vi "Port D_A Output Level.vi"(7 "Read Value? (F)":bool, 8 "error in (no error)":errorcluster, 9 "Port Output Level (0.000 V)":dbl format="%.3g", 10 "Port (1)":T1=enum."1", 11 "VISA resource name":refnum<visa-resource-name>) -> (0 "error out":errorcluster, 1 "Port Output Level":dbl format="%.3g", 3 "VISA resource name out":refnum<visa-resource-name>)   [LabVIEW 2013, in "SRS SR400.lvlib"]
doc: "<B>PL i { ,v }</B>\n\nThe PL command sets and reads thePORT1 and PORT2 output levels. i=1 or 2 to select PORT1 or PORT 2 and is required. If v is included, the output level is set to v Volts where -10.000 <= v <= 10.000. The resolution is 0.005 V (5 mV). If v is absent, the output level is returned. If the Port output mode is SCAN, the PL command sets and reads the starting value of the level. Changing the level during a scan will cause the level to be set to the new value on the next count period. Note that the scan is not reset. Reading the level during a scan always returns the starting value, not the current value."
uses:
  <instrlib>/SRS SR400/SRS SR400.lvlib
  <instrlib>/SRS SR400/Public/Typedefs/Port.ctl
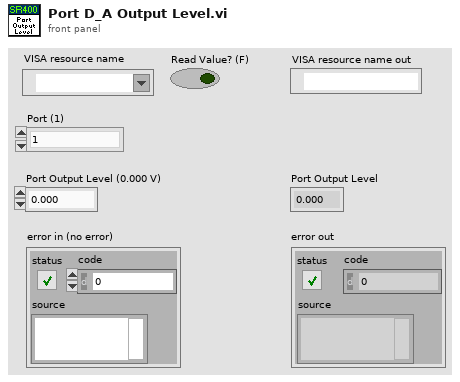
[diagram p1: front panel]
types:
  T1 = typedef "SRS SR400.lvlib/Port.ctl" = enum16{"(not used)", "1", "2"}
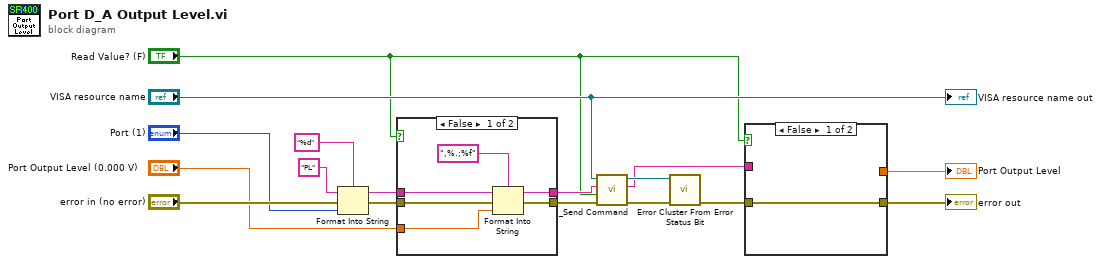
[diagram p0: block diagram]
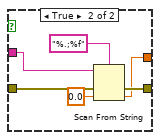
[diagram p2: hidden frame]
diagram:
  n1 = Format Into String(format string="%d", initial string="PL" ("command"), error in="error in (no error)", "Port (1)") -> (resulting string=w15:string, error out=w16:errorcluster)
  n2 = case shown="False" "Read Value? (F)" {
    tunnel: w16 -> [w23 w24]
    tunnel: w15 -> [w18 w25]
    tunnel: "Port Output Level (0.000 V)" -> [w22 _]
    tunnel: [w20 w25] -> w11
    tunnel: [w19 w24] -> w10
    frame False {
      n3 = Format Into String(format string=",%.;%f", initial string=w18, error in=w23, w22) -> (resulting string=w20:string, error out=w19:errorcluster)
    }
    frame True {
    }
  }
  n4 = call <instrlib>:"_Send Command.vi"("error in (no error)"=w10, "Read Value? (F)"="Read Value? (F)", "Command"=w11, "VISA resource name"="VISA resource name") -> ("error out"=w7:errorcluster, "Response"=w4:string, "VISA resource name out"=w8:refnum<visa-resource-name>)  [unwired: 5 out]
  n5 = call <instrlib>:"Error Cluster From Error Status Bit.vi"("error in (no error)"=w7, "VISA resource name"=w8) -> ("error out"=w6:errorcluster)  [unwired: 8 in, 1 out]
  n6 = case shown="False" "Read Value? (F)" {
    tunnel: w6 -> [w26 w32]
    tunnel: [w26 w31] -> w5
    tunnel: w4 -> [_ w30]
    tunnel: [_ w27] -> w3
    frame False {
    }
    frame True {
      n7 = Scan From String(format string="%.;%f", input string=w30, error in=w32, default 1=0.0 ("default value 1")) -> (error out=w31:errorcluster, output 1=w27:dbl)  [unwired: 1 in, 2 out]
    }
  }
  "error out" <- w5
  "Port Output Level" <- w3
  "VISA resource name out" <- "VISA resource name"
